vi "Motor with Encoder - DrH Test v3.vi"() -> ()   [LabVIEW 2016]
doc: "This example shows how to move a motor connected to an encoder and a wheel, and then read information about the system from an encoder.\n\nThis is an example of how to use feedback (from the encoder) to create an open loop system. If some control method was used, for example using PID, a closed loop system could be created.\n\nThis example expects a USB cable connected from your development PC to the Type B USB Jack (next to the power input) on the roboRIO.\n\nThis example requires the Driver Station to be running with Teleoperated Enabled."
uses:
  <vilib>/Rock Robotics/SystemInterfaces/DIO/FPGA_DIOChannel.ctl
  <vilib>/Rock Robotics/WPI/Encoder/WPI_EncoderType.ctl
  <vilib>/Rock Robotics/SystemInterfaces/DIO/FPGA_DIOPWMChannel.ctl
  <vilib>/Rock Robotics/WPI/Counter/WPI_CounterDigitalInputToDigitalSource.vi
  <vilib>/Rock Robotics/WPI/MotorControl/WPI_MotorControlOpen SPARK.vi
panel:
  in  "milliseconds to wait":u32=100
  out "Loop Time (s)":dbl format="%_6f"
  out "Encoder Rate (RPM) 2":dbl=1324.567
  out "XY Graph":cluster{dbl[], dbl[]}[](graph)
  out "Waveform Chart":dbl(graph)
  in  "Motor Speed (-1 to 1)":dbl(slide) step=0.1 scale=-1.0..1.0
  in  "Motor PWM Channel":T1=enum."PWM 2"
  in  "Number Samples to Average":u8=1 min=1 max=128
  in  "Invert Direction":bool
  in  "Decoding Type":T2=enum."4x"
  in  "DistancePerCount (deg)":dbl=0.351563
  in  "Encoder B Channel":T3=enum."DIO 1"
  in  "Encoder A Channel":T3
  out "Encoder Rate (deg/sec)":dbl
  in  "Minimum Rate":dbl=20.0
  in  "Stop":bool
  out "Encoder Alarm Status":string="Encoder Stopped"
  out "Encoder Direction":string="Forward"
  # "These can be set while running."
  # "Output information."
  # "Set these inputs before running."
  # "This example requires the Driver Station to be running with Teleoperated Enabled."
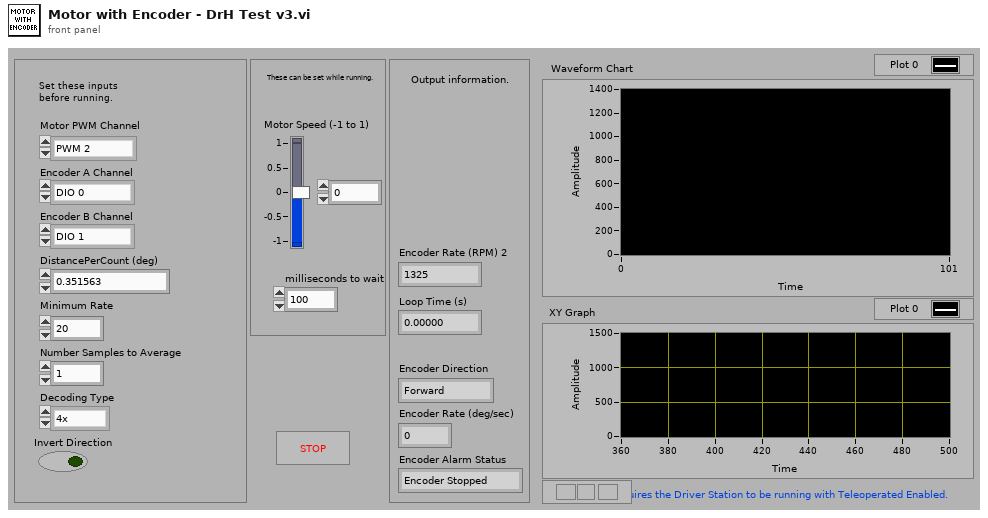
[diagram p1: front panel]
types:
  T1 = typedef "FPGA_DIOPWMChannel.ctl" = enum8{"PWM 0", "PWM 1", "PWM 2", "PWM 3", "PWM 4", "PWM 5", "PWM 6", "PWM 7", "PWM 8", "PWM 9", "PWM MXP 0", "PWM MXP 1", "PWM MXP 2", "PWM MXP 3", "PWM MXP 4", "PWM MXP 5", "PWM MXP 6", "PWM MXP 7", "PWM MXP 8", "PWM MXP 9", "Invalid"}
  T2 = typedef "WPI_EncoderType.ctl" = enum16{"1x", "2x", "4x"}
  T3 = typedef "FPGA_DIOChannel.ctl" = enum8{"DIO 0", "DIO 1", "DIO 2", "DIO 3", "DIO 4", "DIO 5", "DIO 6", "DIO 7", "DIO 8", "DIO 9", "DIO MXP 0", "DIO MXP 1", "DIO MXP 2", "DIO MXP 3", "DIO MXP 4", "DIO MXP 5", "DIO MXP 6", "DIO MXP 7", "DIO MXP 8", "DIO MXP 9", "DIO MXP 10", "DIO MXP 11", "DIO MXP 12", "DIO MXP 13", "DIO MXP 14", "DIO MXP 15", "SPI Port CS1", "SPI Port CS2", "SPI Port CS3", "SPI Port MISO", "SPI Port MOSI", "Invalid"}
  T4 = typedef "WPI_MotorControlDeviceRef.ctl" = cluster{"DeviceStatus":errorcluster, "Type":T5, "PWM":cluster{"PWM Channel":T1, "DeadBand":T6}, "CAN":cluster{"Device Number":u8, "SetOutput VI Ref":variant, "GetOutput VI Ref":variant, "Enable VI Ref":variant, "Disable VI Ref":variant, "Data":variant}, "Invert":bool}
  T5 = typedef "WPI_MotorControlType.ctl" = enum16{"PWM", "CAN"}
  T6 = typedef "WPI_PWMDeadband.ctl" = cluster{"Name":string, "maxPositivePwm":i32, "minPositivePwm":i32, "centerPwm":i32, "maxNegativePwm":i32, "minNegativePwm":i32, "angularRange":u16}
  T7 = typedef "WPI_DigitalInputDevRef.ctl" = cluster{"DevStatus":errorcluster, "DIO Channel":T3}
  T8 = typedef "FPGA_CounterEncoderSourceConvertionLVSourceType.ctl" = cluster{"DevStatus":errorcluster, "AnalogTriggerMode?":bool, "DigitalMode":cluster{"DIO Channel":T9}, "AnalogTriggerMode":cluster{"AnalogTriggerIndex":T10, "OutputType":T11}}
  T9 = typedef "FPGA_DIODigitalSourceChannel.ctl" = enum8{"DIO 0", "DIO 1", "DIO 2", "DIO 3", "DIO 4", "DIO 5", "DIO 6", "DIO 7", "DIO 8", "DIO 9", "DIO MXP 0", "DIO MXP 1", "DIO MXP 2", "DIO MXP 3", "DIO MXP 4", "DIO MXP 5", "DIO MXP 6", "DIO MXP 7", "DIO MXP 8", "DIO MXP 9", "DIO MXP 10", "DIO MXP 11", "DIO MXP 12", "DIO MXP 13", "DIO MXP 14", "DIO MXP 15", "Disabled"}
  T10 = typedef "FPGA_AnalogTriggerIndex.ctl" = enum8{"Trig 0", "Trig 1", "Trig 2", "Trig 3", "Trig 4", "Trig 5", "Trig 6", "Trig 7", "Invalid"}
  T11 = typedef "FPGA_AnalogTriggerOutType.ctl" = enum16{"InWindow", "TriggerState", "Rising", "Falling"}
  T12 = typedef "WPI_EncoderDevRef.ctl" = cluster{"DevStatus":errorcluster, "EncoderIndex":T13, "CounterIndex":T14, "DistancePerCount":dbl, "Decoding Type":T2}
  T13 = typedef "FPGA_EncoderIdx.ctl" = enum8{"Enc 0", "Enc 1", "Enc 2", "Enc 3", "Enc 4", "Enc 5", "Enc 6", "Enc 7", "Invalid"}
  T14 = typedef "FPGA_CounterCtrSystemIndex.ctl" = enum8{"Ctr 0", "Ctr 1", "Ctr 2", "Ctr 3", "Ctr 4", "Ctr 5", "Ctr 6", "Ctr 7", "Invalid"}
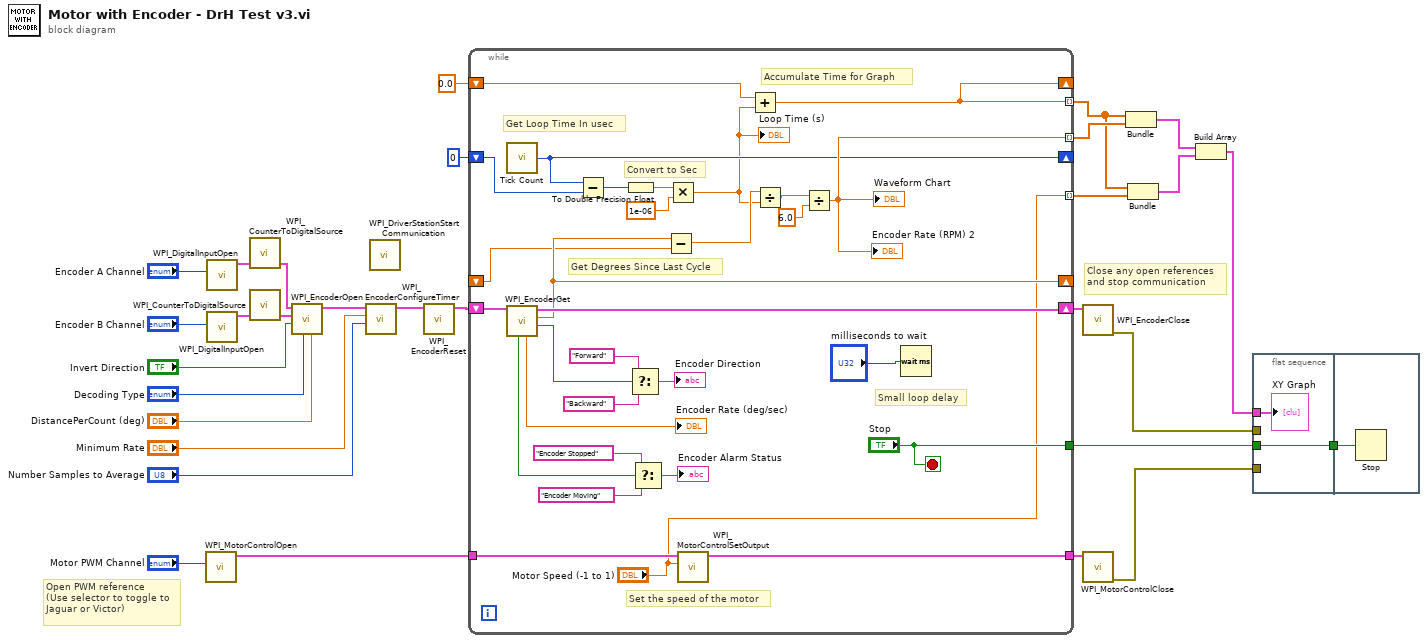
[diagram p0: block diagram]
diagram:
  # "Open PWM reference\n(Use selector to toggle to Jaguar or Victor)"
  # "Close any open references\nand stop communication"
  n1 = call-poly <vilib>:"WPI_MotorControlOpen.vi"("PWM Channel"="Motor PWM Channel") -> ("MotorControlDeviceRef"=w16:T4)  [unwired: 3 in, 7 out]
  n2 = call <vilib>:"WPI_DigitalInputOpen.vi"("DIO Channel"="Encoder A Channel") -> ("DigitalInputDevRef"=w27:T7)  [unwired: 1 in, 9 out]
  n3 = call <vilib>:"WPI_DigitalInputOpen.vi"("DIO Channel"="Encoder B Channel") -> ("DigitalInputDevRef"=w28:T7)  [unwired: 1 in, 9 out]
  n4 = call-poly <vilib>:"WPI_CounterToDigitalSource.vi"("DigitalInputDevRef"=w27) -> ("Digital Source"=w26:T8)  [unwired: 6 out]
  n5 = call-poly <vilib>:"WPI_CounterToDigitalSource.vi"("DigitalInputDevRef"=w28) -> ("Digital Source"=w29:T8)  [unwired: 6 out]
  n6 = call <vilib>:"WPI_EncoderOpen.vi"("DistancePerCount"="DistancePerCount (deg)", "Decoding Type"="Decoding Type", "Invert Direction (False)"="Invert Direction", "BSource"=w29, "ASource"=w26) -> ("EncoderDevRef"=w20:T12)  [unwired: 3 in, 3 out]
  n7 = call <vilib>:"WPI_EncoderConfigureTimer.vi"("Number Samples to Average"="Number Samples to Average", "Minimum Rate"="Minimum Rate", "EncoderDevRef"=w20) -> ("EncoderDevRef"=w12:T12)  [unwired: 1 in, 7 out]
  n8 = call <vilib>:"WPI_DriverStationStart Communication.vi"() -> ()  [unwired: 2 in, 10 out]
  n9 = call <vilib>:"WPI_EncoderReset.vi"("EncoderDevRef"=w12) -> ("EncoderDevRef"=w11:T12)  [unwired: 1 in, 9 out]
  n10 = while {
    shift-right: [w44] -> w30
    shift-left: w11 -> [w48]
    tunnel: ["Stop"] -> w14
    tunnel: w16 -> [w52]
    tunnel: [w51] -> w17
    tunnel: [w45] -> w13 mode=indexing
    tunnel: [w32] -> w7 mode=indexing
    shift-right: [w43] -> _
    shift-left: u32 0 ("Tick Count(uSec)") -> [w42]
    shift-right: [w41] -> _
    shift-left: _ -> [w40]
    shift-right: [w32] -> _
    shift-left: 0.0 ("Tick Count(uSec)") -> [w33]
    tunnel: ["Motor Speed (-1 to 1)"] -> w6 mode=indexing
    stop <- "Stop" stop-if-true
    # "Accumulate Time for Graph"
    # "Get Degrees Since Last Cycle"
    # "Convert to Sec"
    # "Get Loop Time In usec"
    # "Set the speed of the motor"
    # "Small loop delay"
    n11 = call "Tick Count"() -> ("Tick Count(uSec)"=w43:u32)
    n12 = call <vilib>:"WPI_EncoderGet.vi"("EncoderDevRef"=w48) -> ("Direction"=w58:bool, "Distance"=w41:dbl, "EncoderDevRef"=w44:T12, "Rate"=→"Encoder Rate (deg/sec)":dbl, "Stopped"=w57:bool)  [unwired: 1 in, 5 out]
    n13 = Subtract(x=w43, y=w42) -> (x-y=w39:u32)
    n14 = To Double Precision Float(number=w39) -> (double precision float=w37:dbl)
    n15 = Select(t="Forward", s=w58, f="Backward") -> (s? t:f=→"Encoder Direction":string)
    n16 = Select(t="Encoder Stopped", s=w57, f="Encoder Moving") -> (s? t:f=→"Encoder Alarm Status":string)
    n17 = Subtract(x=w41, y=w40) -> (x-y=w36:dbl)
    n18 = Multiply(x=w37, y=1e-06) -> (x*y=w34:dbl)
    "Loop Time (s)" <- w34
    n19 = call <vilib>:"WPI_MotorControlSetOutput.vi"("Output"="Motor Speed (-1 to 1)", "MotorControlDevRef"=w52) -> ("MotorControlDevRef"=w51:T4)  [unwired: 2 in, 7 out]
    n20 = Add(x=w33, y=w34) -> (x+y=w32:dbl)
    n21 = Divide(x=w36, y=w34) -> (x/y=w35:dbl)
    n22 = Divide(x=w35, y=6.0) -> (x/y=w45:dbl)
    "Waveform Chart" <- w45
    "Encoder Rate (RPM) 2" <- w45
    n23 = Wait (ms)(milliseconds to wait="milliseconds to wait") -> ()  [unwired: 1 out]
  }
  n24 = call <vilib>:"WPI_EncoderClose.vi"("EncoderDevRef"=w30) -> ("error out"=w2:errorcluster)  [unwired: 2 in, 8 out]
  n25 = call <vilib>:"WPI_MotorControlClose.vi"("MotorControlDevRef"=w17) -> ("error out"=w1:errorcluster)  [unwired: 1 in, 9 out]
  n26 = Bundle(w7, w13) -> (w5:cluster{dbl[], dbl[]})  [unwired: 1 in]
  n27 = Bundle(w7, w6) -> (w4:cluster{dbl[], dbl[]})  [unwired: 1 in]
  n28 = Build Array(w5, w4) -> (w3:cluster{dbl[], dbl[]}[])
  n29 = flat-sequence {
    tunnel: w14 -> [w62]
    tunnel: [w62] -> w10
    tunnel: w3 -> [w61]
    tunnel: w2 -> [_]
    tunnel: w1 -> [_]
    tunnel: w10 -> [w63]
    frame #0 {
      "XY Graph" <- w61
    }
    frame #1 {
      n30 = Stop(stop? (T)=w63) -> ()
    }
  }
